vi "Configure Bus Source.vi"   [LabVIEW 2015, in "Tektronix 7000 Series.lvlib"]
doc: "Configures Bus settings for an oscilloscope."
uses:
  <instrlib>/Tektronix 7000 Series/Tektronix 7000 Series.lvlib
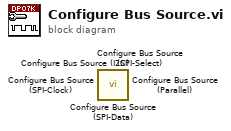
[diagram p0: block diagram]
diagram:
  n1 = call <instrlib>:"Configure Bus Source (SPI-Data).vi"() -> ()  [unwired: 10 in, 2 out]
  n2 = call <instrlib>:"Configure Bus Source (SPI-Select).vi"() -> ()  [unwired: 10 in, 2 out]
  n3 = call <instrlib>:"Configure Bus Source (SPI-Clock).vi"() -> ()  [unwired: 10 in, 2 out]
  n4 = call <instrlib>:"Configure Bus Source (Parallel).vi"() -> ()  [unwired: 10 in, 2 out]
  n5 = call <instrlib>:"Configure Bus Source (I2C).vi"() -> ()  [unwired: 10 in, 2 out]
